vi "mode_natural_freq_check.vi"() -> ()   [LabVIEW 2020]
uses:
  <vilib>/express/express analysis/Spectral/Block/exnSpectralBlock spectral measurements RMS poly.vi
  <vilib>/express/express analysis/Spectral/Block/exnSpectralBlock spectral measurements RMS DDT.vi
  <vilib>/express/express analysis/Spectral/XNode/ExpressSpectralMeasurementsBlockNode.xnode
panel:
  out "error out":errorcluster
  out "task out":refnum<k21>
  in  "device name":tag="Dev1"
  in  "stop (T)":bool=TRUE
  in  "error in":errorcluster
  in  "timeout (s)":dbl=10.0 format="%0.2f"
  in  "number of samples":i32=300000
  in  "rate":dbl=25.0
  out "file location for Time series":path
  out "file location for FFT":path
  out "FFT":dynamicdata(graph)
  out "data":dynamicdata(graph)
  # "FFT"
  # "NI-9234\nNI USB-9162\naccelerometer_J352C33 SN 45481"
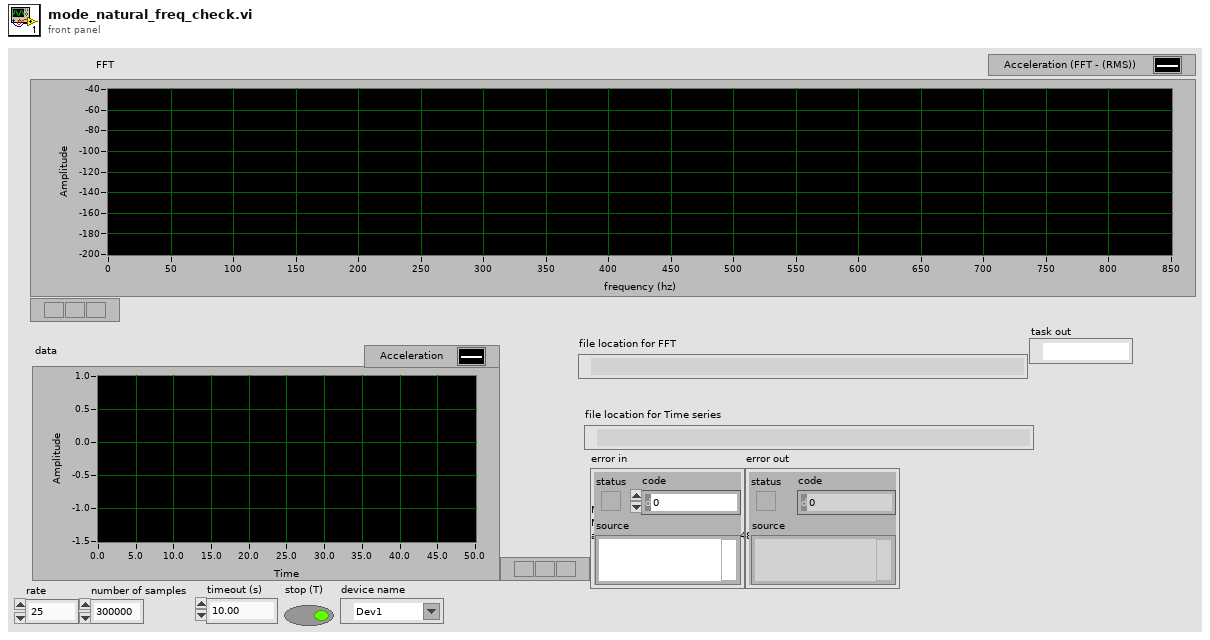
[diagram p1: front panel]
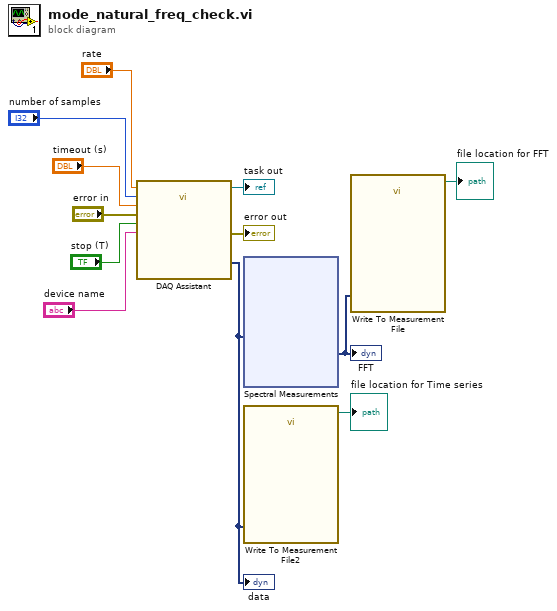
[diagram p0: block diagram]
diagram:
  n1 = call "DAQ Assistant"("rate"="rate", "number of samples"="number of samples", "timeout (s)"="timeout (s)", "error in"="error in", "stop (T)"="stop (T)", "device name"="device name") -> ("task out"=→"task out":refnum<k21>, "data"=w9:dynamicdata, "error out"=→"error out":errorcluster)  [unwired: 11 in]
  "data" <- w9
  n2 = xnode "Spectral Measurements"("Signals"=w9) -> ("FFT - (RMS)"=w11:dynamicdata)  [unwired: 1 in, 2 out]
  "FFT" <- w11
  n3 = call "Write To Measurement File2"("Signals"=w9) -> ("Filename Out"=→"file location for Time series":path)  [unwired: 16 in, 2 out]
  n4 = call "Write To Measurement File"("Signals"=w11) -> ("Filename Out"=→"file location for FFT":path)  [unwired: 16 in, 2 out]
